vi "Lvi Clock Properties.vi"(0 "TaskRef":i32, 11 "error in (no error)":errorcluster) -> (1 "SupSimultaneousClock":bool, 2 "SupIntClock":bool, 3 "MinExtDivider":dbl, 4 "TaskRef out":i32, 6 "MaxFrequency":dbl, 8 "MinFrequency":dbl, 10 "MaxExtDivivder":dbl, 12 "function return":u32(ring), 13 "SupExtClock":bool, 14 "BaseClock":dbl, 15 "error out":errorcluster)   [LabVIEW 2022 SP3, in "DtLvLink.lvlib"]
doc: "Calls directly into the entry points of the DLL of the Data Acq SDK to return information about the clock properties of the device. This VI is used by the higher-level VI, DtOLClock."
uses:
  DtLvLink.lvlib
  <userlib>/LV-Link3/DtLvLink_64.dll
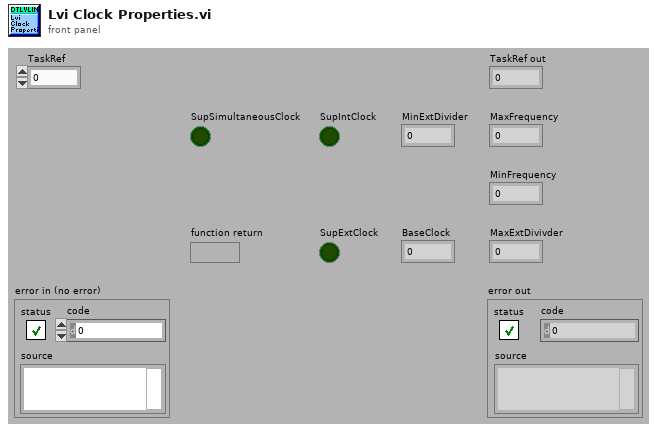
[diagram p1: front panel]
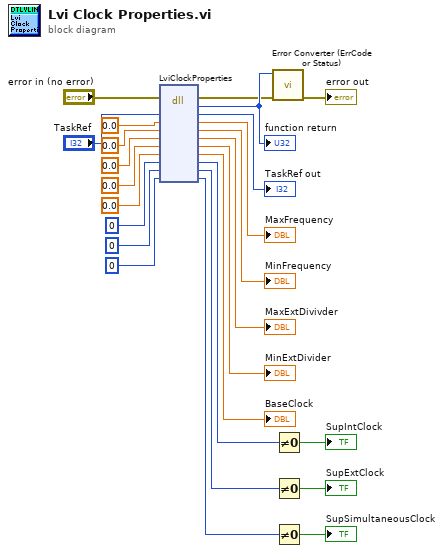
[diagram p0: block diagram]
diagram:
  n1 = dll-call lib="C:/Program Files/National Instruments/LabVIEW 2022/user.lib/LV-Link3/DtLvLink_64.*" fn="LviClockProperties"(error in="error in (no error)", "TaskRef"="TaskRef", "MaxFrequency"=0.0, "MinFrequency"=0.0, "MaxExtDivivder"=0.0, "MinExtDivider"=0.0, "BaseClock"=0.0, "SupIntClock"=u8 0, "SupExtClock"=u8 0, "SupSimultaneousClock"=u8 0) -> (error out=w2:errorcluster, w25:u32, "TaskRef"=→"TaskRef out":i32, "MaxFrequency"=→"MaxFrequency":dbl, "MinFrequency"=→"MinFrequency":dbl, "MaxExtDivivder"=→"MaxExtDivivder":dbl, "MinExtDivider"=→"MinExtDivider":dbl, "BaseClock"=→"BaseClock":dbl, "SupIntClock"=w10:u8, "SupExtClock"=w7:u8, "SupSimultaneousClock"=w4:u8)  [unwired: 2 in, 1 out]
  "function return" <- w25
  n2 = call "Error Converter (ErrCode or Status).vi"("error in (no error)"=w2, "error code"=w25) -> ("error out"=→"error out":errorcluster)  [unwired: 9 in]
  n3 = Not Equal To 0?(x=w10) -> (x != 0?=→"SupIntClock":bool)
  n4 = Not Equal To 0?(x=w7) -> (x != 0?=→"SupExtClock":bool)
  n5 = Not Equal To 0?(x=w4) -> (x != 0?=→"SupSimultaneousClock":bool)
